vi "UTILITY Data Quality Check.vi"(10 "Limit":dbl, 11 "Input Data":dbl) -> (3 "Data Output":dbl)   [LabVIEW 2016]
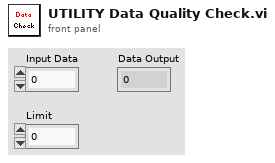
[diagram p1: front panel]
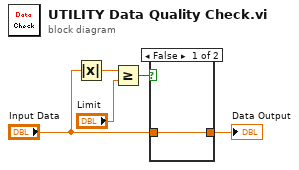
[diagram p0: block diagram]
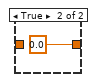
[diagram p2: hidden frame]
diagram:
  n1 = Absolute Value(x="Input Data") -> (abs(x)=w1:dbl)
  n2 = Greater Or Equal?(x=w1, y="Limit") -> (x >= y?=w3:bool)
  n3 = case shown="False" w3 {
    tunnel: [w6 0.0] -> w4
    tunnel: "Input Data" -> [w6 _]
    frame False {
    }
    frame True {
    }
  }
  "Data Output" <- w4
